vi "setDataFIFO.vi"(10 "DataFIFO":refnum<class "IReadU8FIFO.lvclass">, 11 "RTDisplacement in":refnum<class "RTDisplacement.lvclass">) -> (3 "RTDisplacement out":refnum<class "RTDisplacement.lvclass">)   [LabVIEW 2016, in "RTDisplacement.lvlib" / "RTDisplacement.lvclass"]
uses:
  RTDisplacement.lvclass
  Common_RT_FPGA/IReadU8FIFO/IReadU8FIFO.lvclass
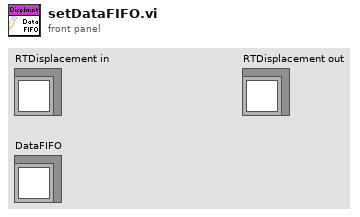
[diagram p1: front panel]
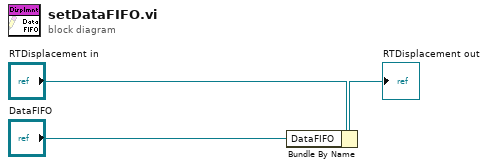
[diagram p0: block diagram]
diagram:
  n1 = Bundle By Name(cluster="RTDisplacement in", "DataFIFO"="DataFIFO") -> (→"RTDisplacement out":refnum<class "RTDisplacement.lvclass">)
